vi "U32ToPixelFormatEnum.vi"(1 "pixel_format_integer":u32 format="%.0x") -> (0 "pixel_format_enum":T1)   [LabVIEW 2026, in "SDL3.lvlib" / "Pixels.lvlib"]
doc: "<B>Summary</B>\nSince LV doesn't allow non contiguous enum values, it must be converted to U32."
uses:
  Pixels.lvlib
  PixelFormat--enum.ctl
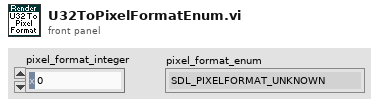
[diagram p1: front panel]
types:
  T1 = typedef "SDL3.lvlib/Pixels.lvlib/PixelFormat--enum.ctl" = enum32{"SDL_PIXELFORMAT_UNKNOWN", "SDL_PIXELFORMAT_INDEX1LSB", "SDL_PIXELFORMAT_INDEX1MSB", "SDL_PIXELFORMAT_INDEX2LSB", "SDL_PIXELFORMAT_INDEX2MSB", "SDL_PIXELFORMAT_INDEX4LSB", "SDL_PIXELFORMAT_INDEX4MSB", "SDL_PIXELFORMAT_INDEX8", "SDL_PIXELFORMAT_RGB332", "SDL_PIXELFORMAT_XRGB4444", "SDL_PIXELFORMAT_XBGR4444", "SDL_PIXELFORMAT_XRGB1555", "SDL_PIXELFORMAT_XBGR1555", "SDL_PIXELFORMAT_ARGB4444", "SDL_PIXELFORMAT_RGBA4444", "SDL_PIXELFORMAT_ABGR4444", "SDL_PIXELFORMAT_BGRA4444", "SDL_PIXELFORMAT_ARGB1555", "SDL_PIXELFORMAT_RGBA5551", "SDL_PIXELFORMAT_ABGR1555", "SDL_PIXELFORMAT_BGRA5551", "SDL_PIXELFORMAT_RGB565", "SDL_PIXELFORMAT_BGR565", "SDL_PIXELFORMAT_RGB24", "SDL_PIXELFORMAT_BGR24", "SDL_PIXELFORMAT_XRGB8888", "SDL_PIXELFORMAT_RGBX8888", "SDL_PIXELFORMAT_XBGR8888", "SDL_PIXELFORMAT_BGRX8888", "SDL_PIXELFORMAT_ARGB8888", "SDL_PIXELFORMAT_RGBA8888", "SDL_PIXELFORMAT_ABGR8888", "SDL_PIXELFORMAT_BGRA8888", "SDL_PIXELFORMAT_XRGB2101010", "SDL_PIXELFORMAT_XBGR2101010", "SDL_PIXELFORMAT_ARGB2101010", "SDL_PIXELFORMAT_ABGR2101010", "SDL_PIXELFORMAT_RGB48", "SDL_PIXELFORMAT_BGR48", "SDL_PIXELFORMAT_RGBA64", "SDL_PIXELFORMAT_ARGB64", "SDL_PIXELFORMAT_BGRA64", "SDL_PIXELFORMAT_ABGR64", "SDL_PIXELFORMAT_RGB48_FLOAT", "SDL_PIXELFORMAT_BGR48_FLOAT", "SDL_PIXELFORMAT_RGBA64_FLOAT", "SDL_PIXELFORMAT_ARGB64_FLOAT", "SDL_PIXELFORMAT_BGRA64_FLOAT", "SDL_PIXELFORMAT_ABGR64_FLOAT", "SDL_PIXELFORMAT_RGB96_FLOAT", "SDL_PIXELFORMAT_BGR96_FLOAT", "SDL_PIXELFORMAT_RGBA128_FLOAT", "SDL_PIXELFORMAT_ARGB128_FLOAT", "SDL_PIXELFORMAT_BGRA128_FLOAT", "SDL_PIXELFORMAT_ABGR128_FLOAT", "SDL_PIXELFORMAT_YV12", "SDL_PIXELFORMAT_IYUV", "SDL_PIXELFORMAT_YUY2", "SDL_PIXELFORMAT_UYVY", "SDL_PIXELFORMAT_YVYU", "SDL_PIXELFORMAT_NV12", "SDL_PIXELFORMAT_NV21", "SDL_PIXELFORMAT_P010", "SDL_PIXELFORMAT_EXTERNAL_OES"}
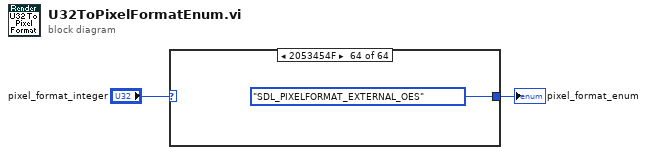
[diagram p0: block diagram]
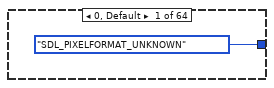
[diagram p2: hidden frame]
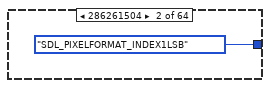
[diagram p3: hidden frame]
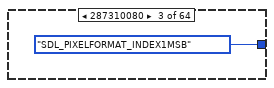
[diagram p4: hidden frame]
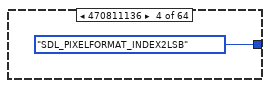
[diagram p5: hidden frame]
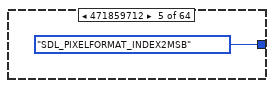
[diagram p6: hidden frame]
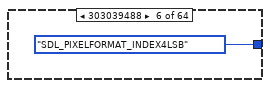
[diagram p7: hidden frame]
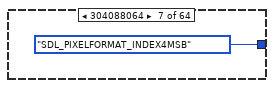
[diagram p8: hidden frame]
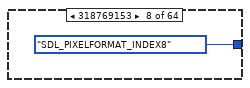
[diagram p9: hidden frame]
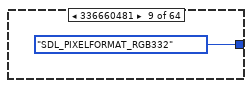
[diagram p10: hidden frame]
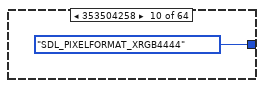
[diagram p11: hidden frame]
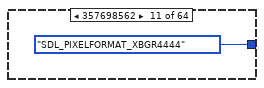
[diagram p12: hidden frame]
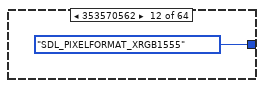
[diagram p13: hidden frame]
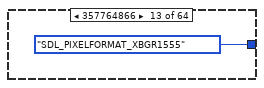
[diagram p14: hidden frame]
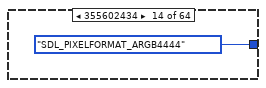
[diagram p15: hidden frame]
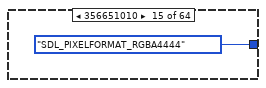
[diagram p16: hidden frame]
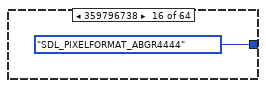
[diagram p17: hidden frame]
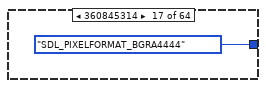
[diagram p18: hidden frame]
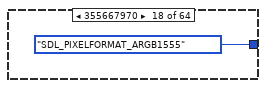
[diagram p19: hidden frame]
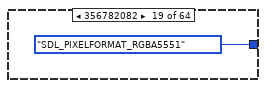
[diagram p20: hidden frame]
diagram:
  n1 = case shown="2053454F" "pixel_format_integer" {
    tunnel: [PixelFormat--enum."SDL_PIXELFORMAT_UNKNOWN" ("pixel_format_enum") PixelFormat--enum."SDL_PIXELFORMAT_INDEX1LSB" ("pixel_format_enum") PixelFormat--enum."SDL_PIXELFORMAT_INDEX1MSB" ("pixel_format_enum") PixelFormat--enum."SDL_PIXELFORMAT_INDEX2LSB" ("pixel_format_enum") PixelFormat--enum."SDL_PIXELFORMAT_INDEX2MSB" ("pixel_format_enum") PixelFormat--enum."SDL_PIXELFORMAT_INDEX4LSB" ("pixel_format_enum") PixelFormat--enum."SDL_PIXELFORMAT_INDEX4MSB" ("pixel_format_enum") PixelFormat--enum."SDL_PIXELFORMAT_INDEX8" ("pixel_format_enum") PixelFormat--enum."SDL_PIXELFORMAT_RGB332" ("pixel_format_enum") PixelFormat--enum."SDL_PIXELFORMAT_XRGB4444" ("pixel_format_enum") PixelFormat--enum."SDL_PIXELFORMAT_XBGR4444" ("pixel_format_enum") PixelFormat--enum."SDL_PIXELFORMAT_XRGB1555" ("pixel_format_enum") PixelFormat--enum."SDL_PIXELFORMAT_XBGR1555" ("pixel_format_enum") PixelFormat--enum."SDL_PIXELFORMAT_ARGB4444" ("pixel_format_enum") PixelFormat--enum."SDL_PIXELFORMAT_RGBA4444" ("pixel_format_enum") PixelFormat--enum."SDL_PIXELFORMAT_ABGR4444" ("pixel_format_enum") PixelFormat--enum."SDL_PIXELFORMAT_BGRA4444" ("pixel_format_enum") PixelFormat--enum."SDL_PIXELFORMAT_ARGB1555" ("pixel_format_enum") PixelFormat--enum."SDL_PIXELFORMAT_RGBA5551" ("pixel_format_enum") PixelFormat--enum."SDL_PIXELFORMAT_ABGR1555" ("pixel_format_enum") PixelFormat--enum."SDL_PIXELFORMAT_BGRA5551" ("pixel_format_enum") PixelFormat--enum."SDL_PIXELFORMAT_RGB565" ("pixel_format_enum") PixelFormat--enum."SDL_PIXELFORMAT_BGR565" ("pixel_format_enum") PixelFormat--enum."SDL_PIXELFORMAT_RGB24" ("pixel_format_enum") PixelFormat--enum."SDL_PIXELFORMAT_BGR24" ("pixel_format_enum") PixelFormat--enum."SDL_PIXELFORMAT_XRGB8888" ("pixel_format_enum") PixelFormat--enum."SDL_PIXELFORMAT_RGBX8888" ("pixel_format_enum") PixelFormat--enum."SDL_PIXELFORMAT_XBGR8888" ("pixel_format_enum") PixelFormat--enum."SDL_PIXELFORMAT_BGRX8888" ("pixel_format_enum") PixelFormat--enum."SDL_PIXELFORMAT_ARGB8888" ("pixel_format_enum") PixelFormat--enum."SDL_PIXELFORMAT_RGBA8888" ("pixel_format_enum") PixelFormat--enum."SDL_PIXELFORMAT_ABGR8888" ("pixel_format_enum") PixelFormat--enum."SDL_PIXELFORMAT_BGRA8888" ("pixel_format_enum") PixelFormat--enum."SDL_PIXELFORMAT_XRGB2101010" ("pixel_format_enum") PixelFormat--enum."SDL_PIXELFORMAT_XBGR2101010" ("pixel_format_enum") PixelFormat--enum."SDL_PIXELFORMAT_ARGB2101010" ("pixel_format_enum") PixelFormat--enum."SDL_PIXELFORMAT_ABGR2101010" ("pixel_format_enum") PixelFormat--enum."SDL_PIXELFORMAT_RGB48" ("pixel_format_enum") PixelFormat--enum."SDL_PIXELFORMAT_BGR48" ("pixel_format_enum") PixelFormat--enum."SDL_PIXELFORMAT_RGBA64" ("pixel_format_enum") PixelFormat--enum."SDL_PIXELFORMAT_ARGB64" ("pixel_format_enum") PixelFormat--enum."SDL_PIXELFORMAT_BGRA64" ("pixel_format_enum") PixelFormat--enum."SDL_PIXELFORMAT_ABGR64" ("pixel_format_enum") PixelFormat--enum."SDL_PIXELFORMAT_RGB48_FLOAT" ("pixel_format_enum") PixelFormat--enum."SDL_PIXELFORMAT_BGR48_FLOAT" ("pixel_format_enum") PixelFormat--enum."SDL_PIXELFORMAT_RGBA64_FLOAT" ("pixel_format_enum") PixelFormat--enum."SDL_PIXELFORMAT_ARGB64_FLOAT" ("pixel_format_enum") PixelFormat--enum."SDL_PIXELFORMAT_BGRA64_FLOAT" ("pixel_format_enum") PixelFormat--enum."SDL_PIXELFORMAT_ABGR64_FLOAT" ("pixel_format_enum") PixelFormat--enum."SDL_PIXELFORMAT_RGB96_FLOAT" ("pixel_format_enum") PixelFormat--enum."SDL_PIXELFORMAT_BGR96_FLOAT" ("pixel_format_enum") PixelFormat--enum."SDL_PIXELFORMAT_RGBA128_FLOAT" ("pixel_format_enum") PixelFormat--enum."SDL_PIXELFORMAT_ARGB128_FLOAT" ("pixel_format_enum") PixelFormat--enum."SDL_PIXELFORMAT_BGRA128_FLOAT" ("pixel_format_enum") PixelFormat--enum."SDL_PIXELFORMAT_ABGR128_FLOAT" ("pixel_format_enum") PixelFormat--enum."SDL_PIXELFORMAT_YV12" ("pixel_format_enum") PixelFormat--enum."SDL_PIXELFORMAT_IYUV" ("pixel_format_enum") PixelFormat--enum."SDL_PIXELFORMAT_YUY2" ("pixel_format_enum") PixelFormat--enum."SDL_PIXELFORMAT_UYVY" ("pixel_format_enum") PixelFormat--enum."SDL_PIXELFORMAT_YVYU" ("pixel_format_enum") PixelFormat--enum."SDL_PIXELFORMAT_NV12" ("pixel_format_enum") PixelFormat--enum."SDL_PIXELFORMAT_NV21" ("pixel_format_enum") PixelFormat--enum."SDL_PIXELFORMAT_P010" ("pixel_format_enum") PixelFormat--enum."SDL_PIXELFORMAT_EXTERNAL_OES" ("pixel_format_enum")] -> w2
    frame 0, Default {
    }
    frame 286261504 {
    }
    frame 287310080 {
    }
    frame 470811136 {
    }
    frame 471859712 {
    }
    frame 303039488 {
    }
    frame 304088064 {
    }
    frame 318769153 {
    }
    frame 336660481 {
    }
    frame 353504258 {
    }
    frame 357698562 {
    }
    frame 353570562 {
    }
    frame 357764866 {
    }
    frame 355602434 {
    }
    frame 356651010 {
    }
    frame 359796738 {
    }
    frame 360845314 {
    }
    frame 355667970 {
    }
    frame 356782082 {
    }
    frame 359862274 {
    }
    frame 360976386 {
    }
    frame 353701890 {
    }
    frame 357896194 {
    }
    frame 386930691 {
    }
    frame 390076419 {
    }
    frame 370546692 {
    }
    frame 371595268 {
    }
    frame 374740996 {
    }
    frame 375789572 {
    }
    frame 372645892 {
    }
    frame 373694468 {
    }
    frame 376840196 {
    }
    frame 377888772 {
    }
    frame 370614276 {
    }
    frame 374808580 {
    }
    frame 372711428 {
    }
    frame 376905732 {
    }
    frame 403714054 {
    }
    frame 406859782 {
    }
    frame 404766728 {
    }
    frame 405815304 {
    }
    frame 407912456 {
    }
    frame 408961032 {
    }
    frame 437268486 {
    }
    frame 440414214 {
    }
    frame 438321160 {
    }
    frame 439369736 {
    }
    frame 441466888 {
    }
    frame 442515464 {
    }
    frame 454057996 {
    }
    frame 457203724 {
    }
    frame 455114768 {
    }
    frame 456163344 {
    }
    frame 458260496 {
    }
    frame 459309072 {
    }
    frame 842094169 {
    }
    frame 1448433993 {
    }
    frame 844715353 {
    }
    frame 1498831189 {
    }
    frame 1431918169 {
    }
    frame 842094158 {
    }
    frame 825382478 {
    }
    frame 808530000 {
    }
    frame 542328143 {
    }
  }
  "pixel_format_enum" <- w2
